vi "PH_Beckhoff.PC set Value.vi"(0 "i ref in":refnum<vi>, 2 "call cluster":T1={"Object"="", "Selector"="", "CallType"=enum."synchronous", "Async Object"="", "Async Selector"="", "Data Descriptor"="", "Data"=[], "Error #"=0, "Expire"=0}, 5 "error in":errorcluster) -> (14 "i ref out":refnum<vi>, 19 "error out":errorcluster)   [LabVIEW 2014, in "PH_Beckhoff.lvlib"]
doc: "This is a pcoc case."
uses:
  PH_Beckhoff.lvlib
  CS_Core/CSSystem/CoreDefs/CoreDefs.call_type.ctl
  CS_Core/BaseProcess/BaseProcess.descriptor string definition.ctl
  CS_Core/CSSystem/CoreDefs/CoreDefs.rawDataType.ctl
  CS_Core/CSSystem/CoreLib/CoreLib.byte array 2 string.vi
  CS_Core/CSSystem/CoreLib/CoreLib.byte array 2 double.vi
  CS_Core/CSSystem/CoreLib/CoreLib.byte array 2 short.vi
  CS_Core/CSSystem/CoreLib/CoreLib.lvlib
  CS_Core/BaseProcess/BaseProcess.lvlib
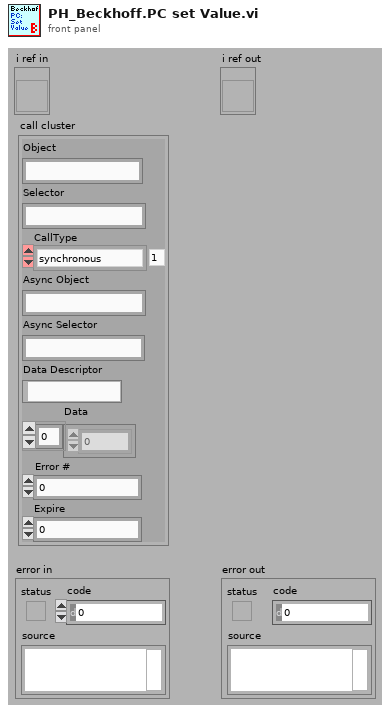
[diagram p1: front panel]
types:
  T1 = typedef "CoreDefs.call_type.ctl" = cluster{"Object":string, "Selector":string, "CallType":enum16{"simple", "synchronous", "asynchronous"}, "Async Object":string, "Async Selector":string, "Data Descriptor":T2, "Data":T3, "Error #":i32, "Expire":u32}
  T2 = typedef "BaseProcess.lvlib/BaseProcess.descriptor string definition.ctl" = string
  T3 = typedef "CoreDefs.rawDataType.ctl" = i8[]
  T4 = typedef "PH_Beckhoff.lvlib/PH_Beckhoff.i attribute.ctl" = cluster{"GUI Refs":T5, "operation?":bool, "Default Prdc Interval":i32, "Connection":T6, "AMS Net ID":T7, "Klemmencluster: # of":T8, "Values":T9, "IP":string, "Description":string, "configured?":bool, "Change Manager":cluster{"Detemination wanted?":bool, "Values changed at":cluster{"Sonderklemmen Inputs":i32[], "Analog Inputs":i32[], "Analog Outputs":i32[], "Digital Inputs":i32[], "Digital Outputs":i32[]}}, "Difference to handle an analog input as change":u32}
  T5 = typedef "PH_Beckhoff.lvlib/PH_Beckhoff.GUI Refs.ctl" = cluster{"ADS Error":refnum<vi>, "Values":refnum<vi>, "configured?":refnum<vi>, "Connection":refnum<vi>, "IP":refnum<vi>, "Prdc Int [ms]":refnum<vi>}
  T6 = typedef "PH_Beckhoff.lvlib/PH_Beckhoff.Connectivity.ctl" = cluster{"DLL?":bool, "Port?":bool, "Client?":bool, "Ping?":bool, "unsuccessful Pings":u32}
  T7 = typedef "Beckhoff - Driver np.lvlib/Beckhoff Access.ctl" = cluster{"DLL path":path, "AMS Net ID":cluster{"1st # of IP":u8, "2nd # of IP":u8, "3rd # of IP":u8, "4th # of IP":u8, "In Port":u8, "Out Port":u8}}
  T8 = typedef "Beckhoff - Driver np.lvlib/Klemmendeclarer.ctl" = cluster{"Offset due to Sonderklemms":u32, "analog Inputs":u32, "analog Outputs":u32, "digital Input Bits":u32, "digital Output Bits":u32}
  T9 = typedef "PH_Beckhoff.lvlib/PH_Beckhoff.Values.ctl" = cluster{"Sonderklemmen Inputs":T10, "Analog Inputs":T11, "Analog Outputs":T13, "Digital Inputs":T14, "Digital Outputs":T15}
  T10 = typedef "PH_Beckhoff.lvlib/PH_Beckhoff.Sonderklemmen Inputs.ctl" = cluster{"Total Length":u32, "Name":string, "Value":u64, "Quality":bool, "Service ID":i32, "Offset":u32, "Length":u32}[]
  T11 = typedef "PH_Beckhoff.lvlib/PH_Beckhoff.Analog Inputs.ctl" = cluster{"Name":string, "Value":u32, "Quality":bool, "Service ID":i32, "Sca Type":T12}[]
  T12 = typedef "PH_Beckhoff.lvlib/PH_Beckhoff.Scaling Type.ctl" = enum16{"none", "0 ... 15 Bit -> 0 ... 5", "0 ... 15 Bit -> 0 ... 10", "0 ... 15 Bit -> 0 ... 25", "0 ... 15 Bit -> 4 ... 20", "0 ... 15 Bit -> 0 ... 1", "0 ... 15 Bit -> 0 ... 20000", "0 ... 15 Bit -> 0 ... 24000"}
  T13 = typedef "PH_Beckhoff.lvlib/PH_Beckhoff.Analog Outputs.ctl" = cluster{"Name":string, "Value":u32, "Quality":bool, "Wanted Value":u32, "Service ID":i32, "Sca Type":T12}[]
  T14 = typedef "PH_Beckhoff.lvlib/PH_Beckhoff.Digital Inputs.ctl" = cluster{"Name":string, "Value":bool, "Quality":bool, "Service ID":i32, "inverted?":bool}[]
  T15 = typedef "PH_Beckhoff.lvlib/PH_Beckhoff.Digital Outputs.ctl" = cluster{"Name":string, "Value":bool, "Quality":bool, "Wanted Value":bool, "Service ID":i32, "inverted?":bool}[]
  T16 = cluster{"Name":string, "Value":u32, "Quality":bool, "Wanted Value":u32, "Service ID":i32, "Sca Type":T12}
  T17 = cluster{"Name":string, "Value":bool, "Quality":bool, "Wanted Value":bool, "Service ID":i32, "inverted?":bool}
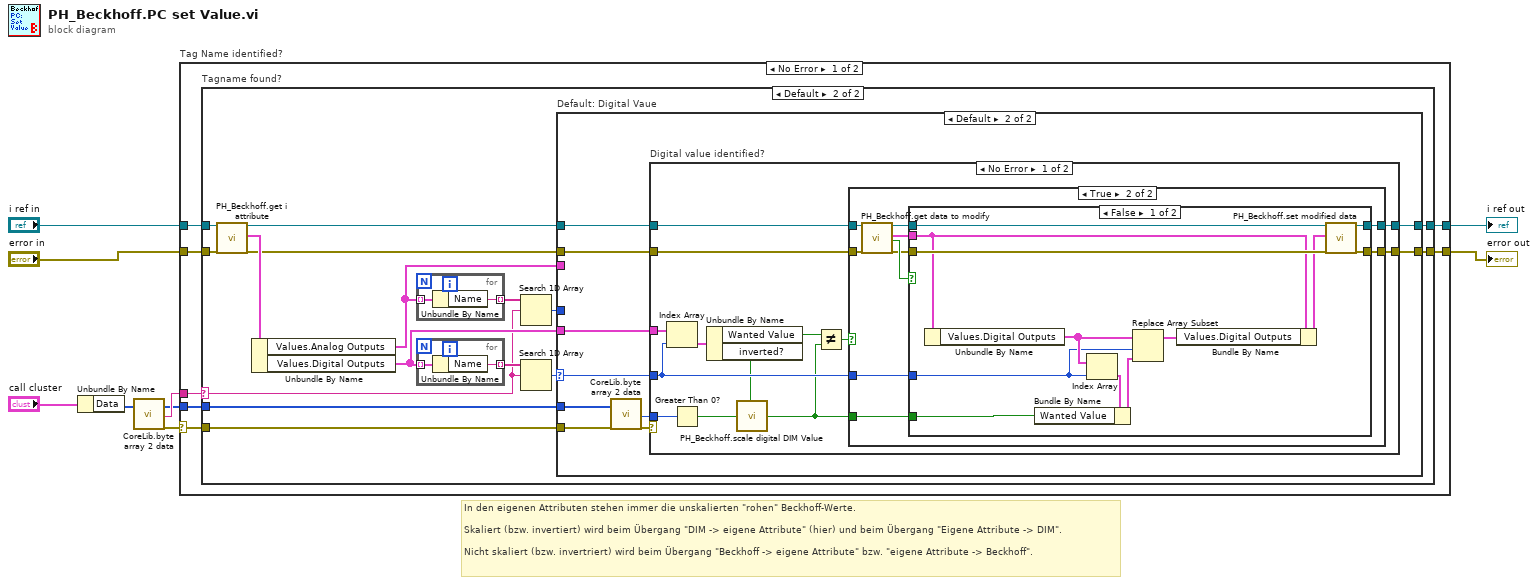
[diagram p0: block diagram]
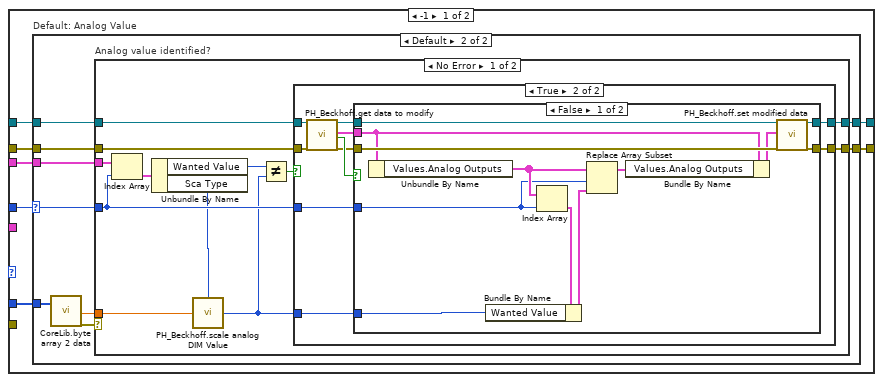
[diagram p3: hidden frame]
diagram:
  # "In den eigenen Attributen stehen immer die unskalierten \"rohen\" Beckhoff-Werte.\n\nSkaliert (bzw. invertiert) wird beim Übergang \"DIM -> eigene Attribute\" (hier) und beim Übergang \"Eigene Attribute -> DIM\".\n\nNicht skaliert (bzw. invertriert) wird beim Übergang \"Beckhoff -> eigene Attribute\" bzw. \"eigene Attribute -> Beckhoff\"."
  n1 = Unbundle By Name("call cluster") -> ("Data"=w5:T3)
  n2 = call-poly "CoreLib.byte array 2 data.vi"("byteArray"=w5) -> ("byteArray out"=w2:T3, "string"=w3:string, "error out"=w1:errorcluster)  [unwired: 16 in]
  n3 = case "Tag Name identified?" shown="No Error" w1 {
    selector: w1 -> [w10 _]
    tunnel: "i ref in" -> [w16 w148]
    tunnel: [w15 w149] -> w8
    tunnel: "error in" -> [w14 w149]
    tunnel: [w13 w148] -> w6
    tunnel: w3 -> [w12 _]
    tunnel: w2 -> [w11 _]
    frame No Error {
      n4 = case "Tagname found?" shown="Default" w12 {
        selector: w12 -> [_ w19]
        tunnel: w16 -> [w18 w32]
        tunnel: [w17 w30] -> w15
        tunnel: w14 -> [w17 w29]
        tunnel: [w18 w28] -> w13
        tunnel: w11 -> [_ w24]
        tunnel: w10 -> [_ w25]
        frame "", "N/A" {
        }
        frame Default {
          n5 = call "PH_Beckhoff.get i attribute.vi"("i ref in"=w32, "error in (no error)"=w29) -> ("i ref out"=w33:refnum<vi>, "i attribute"=w34:T4, "error out"=w31:errorcluster)  [unwired: 15 in]
          n6 = Unbundle By Name(w34) -> ("Values.Analog Outputs"=w21:T13, "Values.Digital Outputs"=w23:T15)
          n7 = for {
            tunnel: w21 -> [w36] mode=indexing
            tunnel: [w35] -> w22 mode=indexing
            n8 = Unbundle By Name(w36) -> ("Name"=w35:string)
          }
          n9 = for {
            tunnel: w23 -> [w147] mode=indexing
            tunnel: [w146] -> w27 mode=indexing
            n10 = Unbundle By Name(w147) -> ("Name"=w146:string)
          }
          n11 = Search 1D Array(1D array=w22, element=w19) -> (index of element=w20:i32)  [unwired: 1 in]
          n12 = Search 1D Array(1D array=w27, element=w19) -> (index of element=w26:i32)  [unwired: 1 in]
          n13 = case "Default: Digital Vaue" shown="Default" w26 {
            selector: w26 -> [_ w99]
            tunnel: w33 -> [w43 w104]
            tunnel: w31 -> [w42 w103]
            tunnel: [w40 w102] -> w30
            tunnel: [w41 w101] -> w28
            tunnel: w23 -> [_ w100]
            tunnel: w25 -> [_ w97]
            tunnel: w24 -> [w38 w96]
            tunnel: w21 -> [w39 _]
            tunnel: w20 -> [w37 _]
            frame -1 {
              n14 = case "Default: Analog Value" shown="Default" w37 {
                selector: w37 -> [_ w46]
                tunnel: w43 -> [w44 w52]
                tunnel: w42 -> [w45 w51]
                tunnel: [w44 w50] -> w41
                tunnel: [w45 w49] -> w40
                tunnel: w39 -> [_ w48]
                tunnel: w38 -> [_ w47]
                frame -1 {
                }
                frame Default {
                  n15 = call-poly "CoreLib.byte array 2 data.vi"("byteArray"=w47) -> ("d64"=w54:dbl, "error out"=w53:errorcluster)  [unwired: 16 in, 1 out]
                  n16 = case "Analog value identified?" shown="No Error" w53 {
                    tunnel: w52 -> [w66 w94]
                    tunnel: w51 -> [w65 w93]
                    tunnel: [w64 w93] -> w49
                    tunnel: [w63 w94] -> w50
                    tunnel: w48 -> [w62 _]
                    tunnel: w46 -> [w59 _]
                    tunnel: w54 -> [w56 _]
                    frame No Error {
                      n17 = Index Array(array=w62, index=w59) -> (element=w61:T16)
                      n18 = Unbundle By Name(w61) -> ("Wanted Value"=w58:u32, "Sca Type"=w57:T12)
                      n19 = call "PH_Beckhoff.scale analog DIM Value.vi"("DIM value"=w56, "Sca Type"=w57) -> ("Beckhoff value"=w55:u32)
                      n20 = Not Equal?(x=w58, y=w55) -> (x != y?=w60:bool)
                      n21 = case shown="True" w60 {
                        tunnel: w66 -> [w68 w78]
                        tunnel: w65 -> [w67 w77]
                        tunnel: [w67 w74] -> w64
                        tunnel: [w68 w72] -> w63
                        tunnel: w59 -> [_ w70]
                        tunnel: w55 -> [_ w69]
                        frame False {
                        }
                        frame True {
                          n22 = call "PH_Beckhoff.get data to modify.vi"("i ref in"=w78, "error in (no error)"=w77) -> ("i ref out"=w71:refnum<vi>, "i attribute"=w75:T4, "timed out"=w76:bool, "error out"=w73:errorcluster)  [unwired: 14 in]
                          n23 = case shown="False" w76 {
                            tunnel: w71 -> [w90 w92]
                            tunnel: [w89 w92] -> w72
                            tunnel: w73 -> [w88 w91]
                            tunnel: [w87 w91] -> w74
                            tunnel: w75 -> [w86 _]
                            tunnel: w70 -> [w82 _]
                            tunnel: w69 -> [w79 _]
                            frame False {
                              n24 = Unbundle By Name(w86) -> ("Values.Analog Outputs"=w83:T13)
                              n25 = Index Array(array=w83, index=w82) -> (element=w81:T16)
                              n26 = Bundle By Name(cluster=w81, "Wanted Value"=w79) -> (w80:T16)
                              n27 = Replace Array Subset(array=w83, new element=w80, index=w82) -> (w84:T13)
                              n28 = Bundle By Name(cluster=w86, "Values.Analog Outputs"=w84) -> (w85:T4)
                              n29 = call "PH_Beckhoff.set modified data.vi"("i ref in"=w90, "i attribute"=w85, "error in (no error)"=w88) -> ("i ref out"=w89:refnum<vi>, "error out"=w87:errorcluster)  [unwired: 15 in]
                            }
                            frame True {
                            }
                          }
                        }
                      }
                    }
                    frame Error {
                    }
                  }
                }
              }
            }
            frame Default {
              n30 = call-poly "CoreLib.byte array 2 data.vi"("byteArray"=w96, "error in (no error)"=w97) -> ("i16"=w98:i16, "error out"=w95:errorcluster)  [unwired: 15 in, 1 out]
              n31 = case "Digital value identified?" shown="No Error" w95 {
                tunnel: w104 -> [w117 w145]
                tunnel: w103 -> [w116 w144]
                tunnel: [w115 w144] -> w102
                tunnel: [w114 w145] -> w101
                tunnel: w100 -> [w113 _]
                tunnel: w99 -> [w110 _]
                tunnel: w98 -> [w109 _]
                frame No Error {
                  n32 = Index Array(array=w113, index=w110) -> (element=w112:T17)
                  n33 = Greater Than 0?(x=w109) -> (x > 0?=w106:bool)
                  n34 = Unbundle By Name(w112) -> ("Wanted Value"=w108:bool, "inverted?"=w107:bool)
                  n35 = call "PH_Beckhoff.scale digital DIM Value.vi"("DIM value"=w106, "inverted?"=w107) -> ("Beckhoff value"=w105:bool)
                  n36 = Not Equal?(x=w108, y=w105) -> (x != y?=w111:bool)
                  n37 = case shown="True" w111 {
                    tunnel: w117 -> [w119 w129]
                    tunnel: w116 -> [w118 w128]
                    tunnel: [w118 w125] -> w115
                    tunnel: [w119 w123] -> w114
                    tunnel: w110 -> [_ w121]
                    tunnel: w105 -> [_ w120]
                    frame False {
                    }
                    frame True {
                      n38 = call "PH_Beckhoff.get data to modify.vi"("i ref in"=w129, "error in (no error)"=w128) -> ("i ref out"=w122:refnum<vi>, "i attribute"=w126:T4, "timed out"=w127:bool, "error out"=w124:errorcluster)  [unwired: 14 in]
                      n39 = case shown="False" w127 {
                        tunnel: w122 -> [w141 w143]
                        tunnel: [w140 w143] -> w123
                        tunnel: w124 -> [w139 w142]
                        tunnel: [w138 w142] -> w125
                        tunnel: w126 -> [w137 _]
                        tunnel: w121 -> [w133 _]
                        tunnel: w120 -> [w130 _]
                        frame False {
                          n40 = Unbundle By Name(w137) -> ("Values.Digital Outputs"=w134:T15)
                          n41 = Index Array(array=w134, index=w133) -> (element=w132:T17)
                          n42 = Bundle By Name(cluster=w132, "Wanted Value"=w130) -> (w131:T17)
                          n43 = Replace Array Subset(array=w134, new element=w131, index=w133) -> (w135:T15)
                          n44 = Bundle By Name(cluster=w137, "Values.Digital Outputs"=w135) -> (w136:T4)
                          n45 = call "PH_Beckhoff.set modified data.vi"("i ref in"=w141, "i attribute"=w136, "error in (no error)"=w139) -> ("i ref out"=w140:refnum<vi>, "error out"=w138:errorcluster)  [unwired: 15 in]
                        }
                        frame True {
                        }
                      }
                    }
                  }
                }
                frame Error {
                }
              }
            }
          }
        }
      }
    }
    frame Error {
    }
  }
  "error out" <- w8
  "i ref out" <- w6
